vi "number-in-counts.vi"(8 "error in (no error)":errorcluster, 9 "Axis Select":u8(slide)=1 min=1 max=4 step=1 scale=1.0..4.0, 10 "unit":enum16{"fs", "ps", "um", "mm", "counts"}(ring), 11 "Number":dbl) -> (0 "error out":errorcluster, 2 "counts":dbl format="%#_18f")   [LabVIEW 2009]
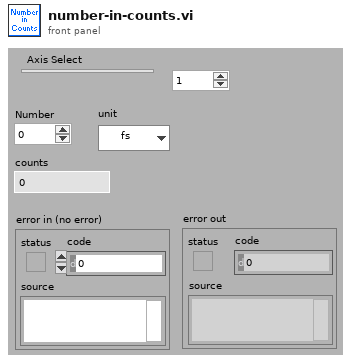
[diagram p1: front panel]
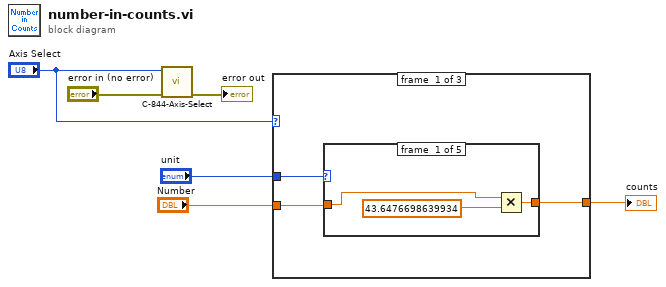
[diagram p0: block diagram]
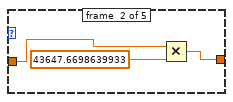
[diagram p2: hidden frame]
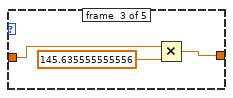
[diagram p3: hidden frame]
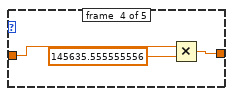
[diagram p4: hidden frame]
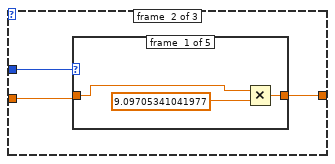
[diagram p6: hidden frame]
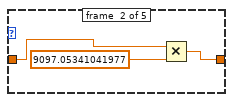
[diagram p7: hidden frame]
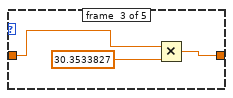
[diagram p8: hidden frame]
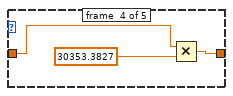
[diagram p9: hidden frame]
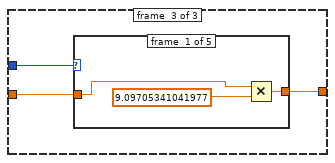
[diagram p11: hidden frame]
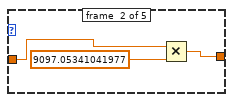
[diagram p12: hidden frame]
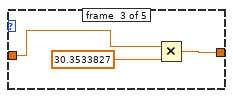
[diagram p13: hidden frame]
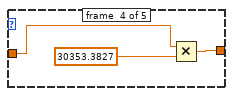
[diagram p14: hidden frame]
diagram:
  n1 = call "C-844-Axis-Select.vi"("error in (no error)"="error in (no error)", "Axis Select"="Axis Select") -> ("error out"=→"error out":errorcluster)  [unwired: 8 in, 1 out]
  n2 = case shown="1, Default" "Axis Select" {
    tunnel: "Number" -> [w7 w25 w39]
    tunnel: "unit" -> [w8 w24 w40]
    tunnel: [w9 w23 w41] -> w4
    frame #0 {
      n3 = case shown="\"counts\"" w8 {
        tunnel: w7 -> [w10 w13 w16 w19 w22]
        tunnel: [w12 w15 w18 w21 w22] -> w9
        frame #0 {
          n4 = Multiply(x=w10, y=43.6476698639934) -> (x*y=w12:dbl)
        }
        frame #1 {
          n5 = Multiply(x=w13, y=43647.6698639933) -> (x*y=w15:dbl)
        }
        frame #2 {
          n6 = Multiply(x=w16, y=145.635555555556) -> (x*y=w18:dbl)
        }
        frame #3 {
          n7 = Multiply(x=w19, y=145635.555555556) -> (x*y=w21:dbl)
        }
        frame #4 {
        }
      }
    }
    frame #1 {
      n8 = case shown="\"fs\", Default" w24 {
        tunnel: w25 -> [w26 w29 w32 w35 w38]
        tunnel: [w28 w31 w34 w37 w38] -> w23
        frame #0 {
          n9 = Multiply(x=w26, y=9.09705341041977) -> (x*y=w28:dbl)
        }
        frame #1 {
          n10 = Multiply(x=w29, y=9097.05341041977) -> (x*y=w31:dbl)
        }
        frame #2 {
          n11 = Multiply(x=w32, y=30.3533827) -> (x*y=w34:dbl)
        }
        frame #3 {
          n12 = Multiply(x=w35, y=30353.3827) -> (x*y=w37:dbl)
        }
        frame #4 {
        }
      }
    }
    frame #2 {
      n13 = case shown="\"ps\"" w40 {
        tunnel: w39 -> [w42 w45 w48 w51 w54]
        tunnel: [w44 w47 w50 w53 w54] -> w41
        frame #0 {
          n14 = Multiply(x=w42, y=9.09705341041977) -> (x*y=w44:dbl)
        }
        frame #1 {
          n15 = Multiply(x=w45, y=9097.05341041977) -> (x*y=w47:dbl)
        }
        frame #2 {
          n16 = Multiply(x=w48, y=30.3533827) -> (x*y=w50:dbl)
        }
        frame #3 {
          n17 = Multiply(x=w51, y=30353.3827) -> (x*y=w53:dbl)
        }
        frame #4 {
        }
      }
    }
  }
  "counts" <- w4
